vi "KE622x -- Get Meas Elements.vi"(0 "Resource In":refnum<visa-resource-name>, 1 "Check For SCPI Errors? (T)":bool=TRUE, 11 "error in (no error)":errorcluster) -> (4 "Resource Out (dupl)":refnum<visa-resource-name>, 8 "Meas Elements To Return":T1={"Timstamp?"=TRUE, "Reading Num?"=TRUE, "Source Value?"=FALSE, "Compliance?"=FALSE, "Average Voltage?"=FALSE}, 15 "error out":errorcluster)   [LabVIEW 2020, in "Keithley 622x.lvlib"]
doc: "Returns the user-specified data fields that will be returned when the trace buffer is read. Note that all fields are _always_ stored -- this VI just indicates the current settings for what will be returned when the buffer is read. Note that this can be changed at any time using the corresponding set VI. For example, the user can read the same buffer contents twice, specifiying different fields to return each time."
uses:
  Keithley 622x.lvlib
  Typedefs/KE622x -- Optional Meas Elements.ctl
panel:
  # "*** NOTE:  \"Average Voltage\"\nis only available for Differential\nConductance measurements."
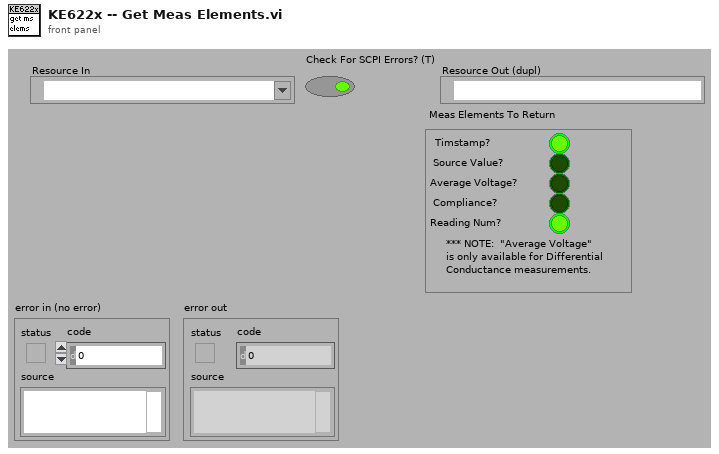
[diagram p1: front panel]
types:
  T1 = typedef "Keithley 622x.lvlib/KE622x -- Optional Meas Elements.ctl" = cluster{"Timstamp?":bool, "Reading Num?":bool, "Source Value?":bool, "Compliance?":bool, "Average Voltage?":bool}
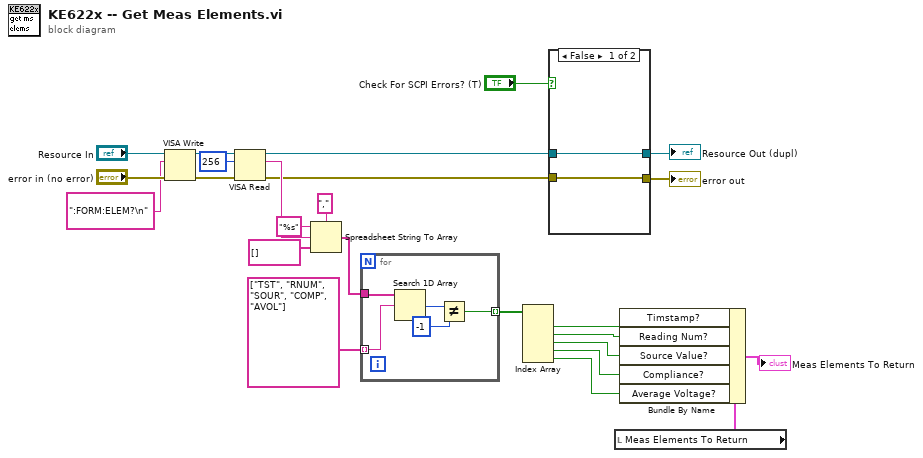
[diagram p0: block diagram]
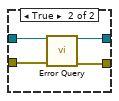
[diagram p2: hidden frame]
diagram:
  n1 = VISA Write(VISA resource name="Resource In", write buffer=":FORM:ELEM?\n" ("format string"), error in (no error)="error in (no error)") -> (VISA resource name out=w19:refnum<visa-resource-name>, error out=w18:errorcluster)  [unwired: 1 out]
  n2 = VISA Read(VISA resource name=w19, byte count=u32 256, error in (no error)=w18) -> (VISA resource name out=w16:refnum<visa-resource-name>, read buffer=w13:string, error out=w6:errorcluster)  [unwired: 1 out]
  n3 = Spreadsheet String To Array(delimiter (Tab)=",", format string="%s", spreadsheet string=w13, array type (2D Dbl)=string[] []) -> (array=w9:string[])
  n4 = for {
    tunnel: w9 -> [w30]
    tunnel: string[] ["TST", "RNUM", "SOUR", "COMP", "AVOL"] -> [w29] mode=indexing
    tunnel: [w26] -> w7 mode=indexing
    n5 = Search 1D Array(1D array=w30, element=w29) -> (index of element=w28:i32)  [unwired: 1 in]
    n6 = Not Equal?(x=w28, y=-1) -> (x != y?=w26:bool)
  }
  n7 = Index Array(array=w7) -> (element #1=w5:bool, element #2=w4:bool, element #3=w3:bool, element #4=w2:bool, element #5=w1:bool)  [unwired: 5 in]
  n8 = case shown="False" "Check For SCPI Errors? (T)" {
    tunnel: w16 -> [w32 w36]
    tunnel: w6 -> [w31 w35]
    tunnel: [w31 w34] -> w21
    tunnel: [w32 w33] -> w22
    frame False {
    }
    frame True {
      n9 = call "Error Query.vi"("VISA Resource In"=w36, "error in (no error)"=w35) -> ("VISA Resource Out (dupl)"=w33:refnum<visa-resource-name>, "error out"=w34:errorcluster)  [unwired: 10 in, 2 out]
    }
  }
  "Resource Out (dupl)" <- w22
  "error out" <- w21
  n10 = local read "Meas Elements To Return"() -> (w15:T1)
  n11 = Bundle By Name(cluster=w15, "Timstamp?"=w5, "Reading Num?"=w4, "Source Value?"=w3, "Compliance?"=w2, "Average Voltage?"=w1) -> (→"Meas Elements To Return":T1)
